vi "WriteTable.vi"(8 "error in (no error)":errorcluster, 10 "Table in":refnum<vi>, 11 "HealthCheck in":refnum<class "HealthCheck.lvclass">) -> (0 "error out":errorcluster, 3 "HealthCheck out":refnum<class "HealthCheck.lvclass">)   [LabVIEW 2018, in "HealthCheck.lvclass"]
uses:
  HealthCheck.lvclass
  <vilib>/Utility/miscctls.llb/LVRowAndColumnTypeDef.ctl
  HealthCheck.lvclass/HealthCheck.ctl
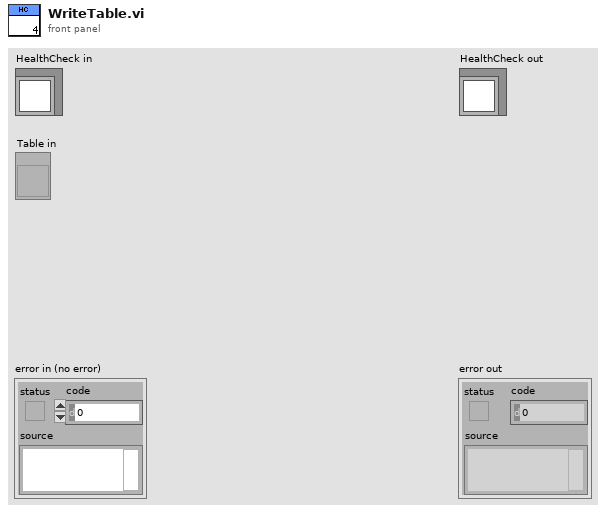
[diagram p1: front panel]
types:
  T1 = typedef "LVRowAndColumnTypeDef.ctl" = cluster{"Row":i32, "Column":i32}
  T2 = typedef "HealthCheck.lvclass/DataEntry_TypeDef.ctl" = cluster{"Data Name":string, "Units":string, "Minimum Value":string, "Maximum Value":string, "Actual Value":string, "Precision":i16}
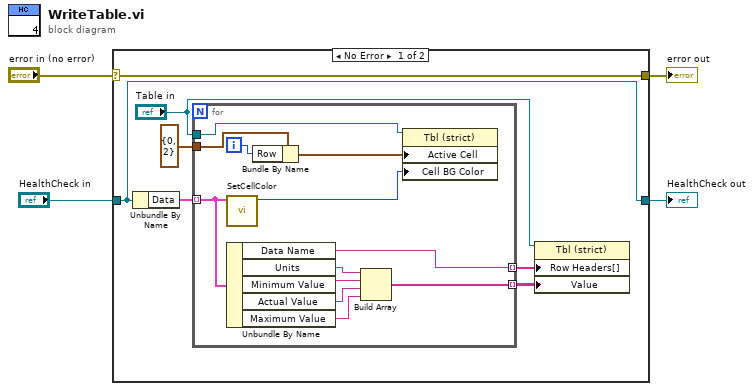
[diagram p0: block diagram]
diagram:
  n1 = case shown="No Error" "error in (no error)" {
    selector: "error in (no error)" -> [w11 w25]
    tunnel: [w11 w25] -> w3
    tunnel: [w10 w24] -> w1
    tunnel: "HealthCheck in" -> [w10 w24]
    frame No Error {
      n2 = Unbundle By Name(w10) -> ("Data"=w9:T2[])
      n3 = for {
        tunnel: w9 -> [w18] mode=indexing
        tunnel: [w19] -> w8 mode=indexing
        tunnel: "Table in" -> [w17]
        tunnel: T1 {"Row"=0, "Column"=2} ("Active Cell:Active Cell") -> [w15]
        tunnel: [w12] -> w5 mode=indexing
        i -> [w13]
        n4 = call "SetCellColor.vi"("Sensor Info"=w18) -> ("Color"=w16:u32)  [unwired: 10 in]
        n5 = Unbundle By Name(w18) -> ("Data Name"=w12:string, "Units"=w23:string, "Minimum Value"=w22:string, "Actual Value"=w21:string, "Maximum Value"=w20:string)
        n6 = Bundle By Name(cluster=w15, "Row"=w13) -> (w14:T1)
        n7 = Build Array(w23, w22, w21, w20) -> (w19:string[])
        n8 = property class="Tbl (strict)"(reference=w17, "Active Cell"=w14, "Cell BG Color"=w16) -> ()  [unwired: 1 in, 2 out]
      }
      n9 = property class="Tbl (strict)"(reference="Table in", "Row Headers[]"=w5, "Value"=w8) -> ()  [unwired: 1 in, 2 out]
    }
    frame Error {
    }
  }
  "error out" <- w3
  "HealthCheck out" <- w1
